vi "MWC.vi"() -> ()   [LabVIEW 2010]
doc: "This is the Target Temperature Monitoring module (TTM).\nIts job is to read all temperature measurement devices and report back the information."
panel:
  in  "Case Constant\n(See Context Help)":bool
  in  "Read HP":bool
  in  "Read FM":bool
  in  "Read Bellows":bool
  in  "Read EIP":bool=TRUE
  out "MWC Message Type":T1(ring)=enum."GenEvent="
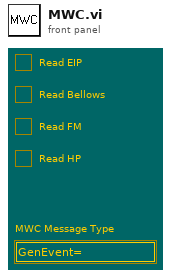
[diagram p1: front panel]
types:
  T1 = enum16{"Bad Message", "No Message", "FMAmplitude=", "FMOffset=", "Tune=", "Switch=", "GenEvent=", "Read", "Ping=", "Stop"}
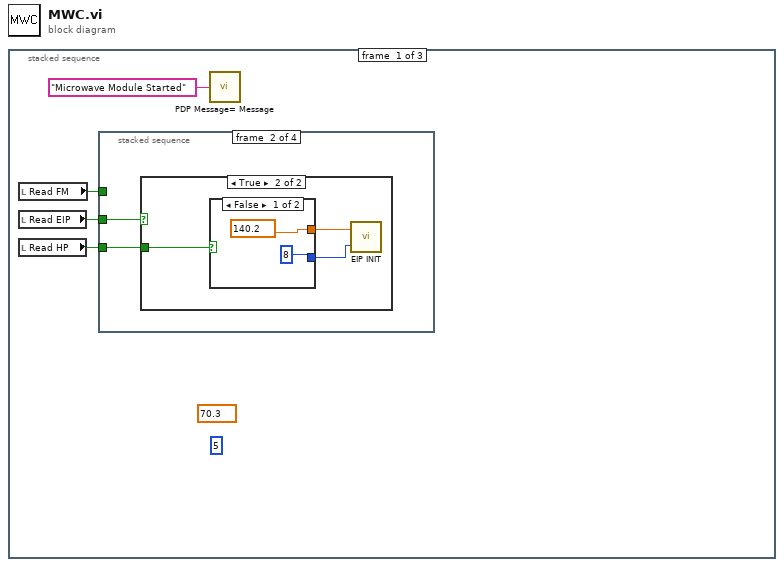
[diagram p0: block diagram]
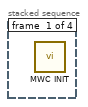
[diagram p2: hidden frame]
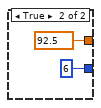
[diagram p4: hidden frame]
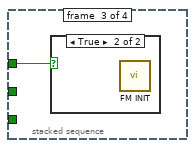
[diagram p5: hidden frame]
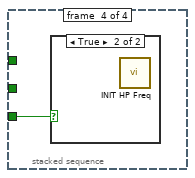
[diagram p7: hidden frame]
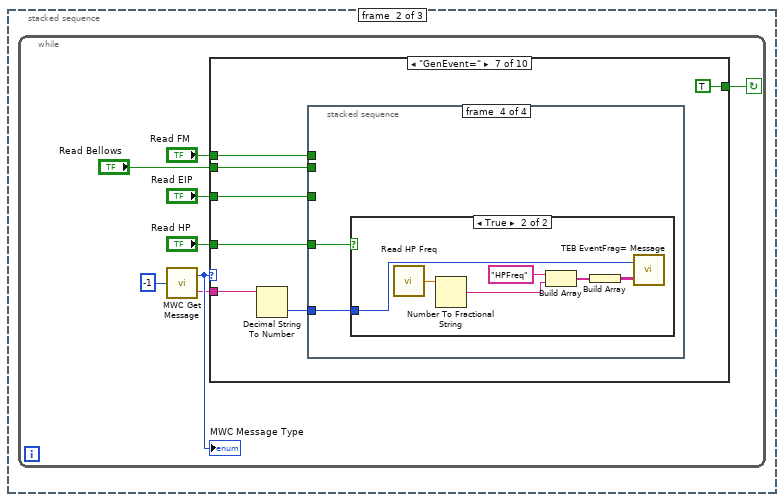
[diagram p9: hidden frame]
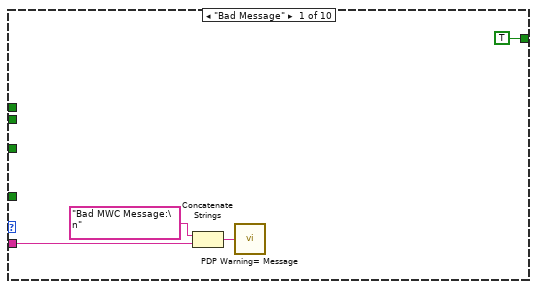
[diagram p10: hidden frame]
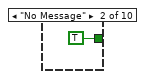
[diagram p11: hidden frame]
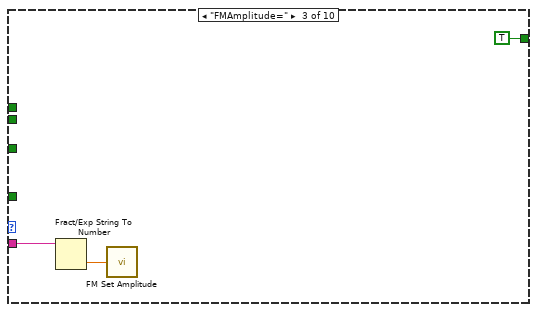
[diagram p12: hidden frame]
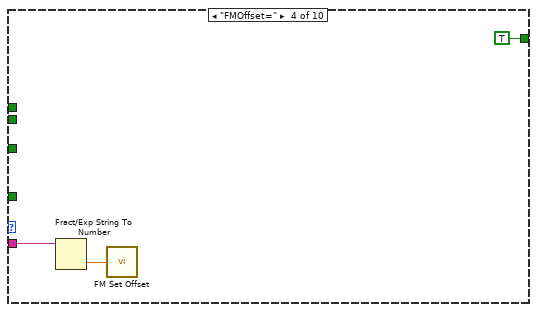
[diagram p13: hidden frame]
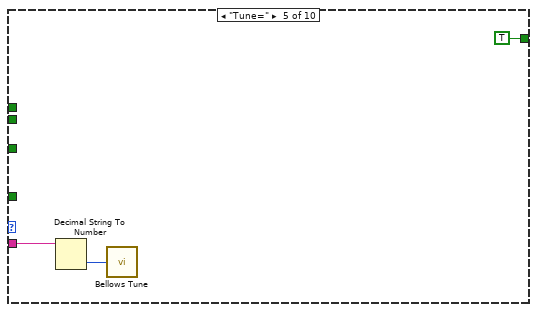
[diagram p14: hidden frame]
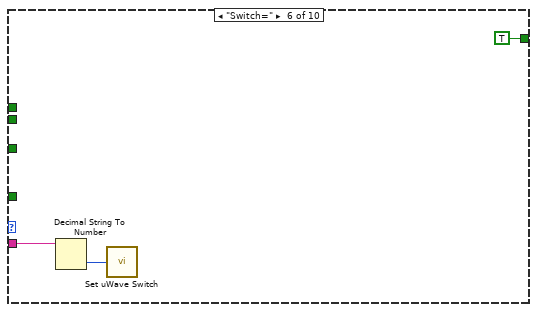
[diagram p15: hidden frame]
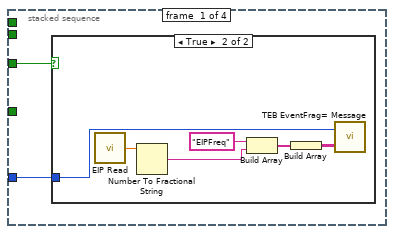
[diagram p16: hidden frame]
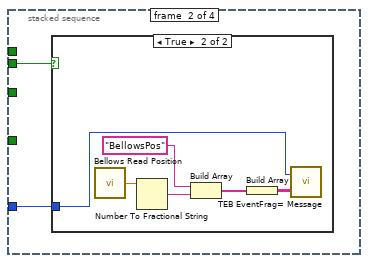
[diagram p18: hidden frame]
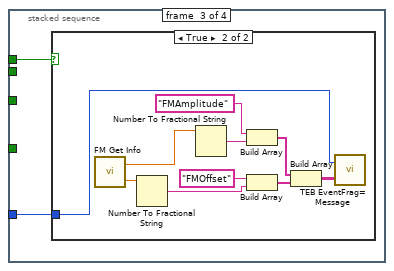
[diagram p20: hidden frame]
diagram:
  n1 = stacked-sequence {
    frame #0 {
      (unwired) 5 ("Subband")
      (unwired) 70.3 ("Center Freq (GHz)")
      n2 = local read "Read FM"() -> (w2:bool)
      n3 = local read "Read EIP"() -> (w1:bool)
      n4 = local read "Read HP"() -> (w3:bool)
      n5 = stacked-sequence {
        tunnel: w2 -> [_ _ w14 _]
        tunnel: w3 -> [_ w5 _ w15]
        tunnel: w1 -> [_ w6 _ _]
        frame #0 {
          n6 = call "MWC INIT.vi"() -> ()  [unwired: 1 in]
        }
        frame #1 {
          n7 = case shown="True" w6 {
            tunnel: w5 -> [_ w7]
            frame False {
            }
            frame True {
              n8 = case shown="False" w7 {
                tunnel: [140.2 ("Center Freq (GHz)") 92.5 ("Center Freq (GHz)")] -> w9
                tunnel: [8 ("Subband") 6 ("Subband")] -> w8
                frame False {
                }
                frame True {
                }
              }
              n9 = call "EIP INIT.vi"("Subband"=w8, "Center Freq (GHz)"=w9) -> ()
            }
          }
        }
        frame #2 {
          n10 = case shown="True" w14 {
            frame False {
            }
            frame True {
              n11 = call "FM INIT.vi"() -> ()  [unwired: 1 in]
            }
          }
        }
        frame #3 {
          n12 = case shown="True" w15 {
            frame False {
            }
            frame True {
              n13 = call "INIT HP Freq.vi"() -> ()  [unwired: 1 in]
            }
          }
        }
      }
      n14 = call "PDP Message= Message.vi"("Message"="Microwave Module Started") -> ()
    }
    frame #1 {
      n15 = while {
        stop <- w23 continue-if-true
        n16 = call "MWC Get Message.VI"("Timeout ms (-1)"=-1) -> ("MWC Message Type"=w22:T1, "Text"=w21:string)
        "MWC Message Type" <- w22
        n17 = case shown="\"GenEvent=\"" w22 {
          tunnel: w21 -> [w27 _ w30 w33 w36 w39 w47 _ w90 _]
          tunnel: [TRUE TRUE TRUE TRUE TRUE TRUE TRUE TRUE TRUE FALSE] -> w23
          tunnel: "Read EIP" -> [_ _ _ _ _ _ w44 _ _ _]
          tunnel: "Read Bellows" -> [_ _ _ _ _ _ w43 _ _ _]
          tunnel: "Read FM" -> [_ _ _ _ _ _ w42 _ _ _]
          tunnel: "Read HP" -> [_ _ _ _ _ _ w41 _ _ _]
          frame "Bad Message" {
            n18 = Concatenate Strings("Bad MWC Message:\n", w27) -> (w25:string)
            n19 = call "PDP Warning= Message.vi"("Message"=w25) -> ()
          }
          frame "No Message" {
          }
          frame "FMAmplitude=" {
            n20 = Fract/Exp String To Number(string=w30) -> (number=w29:dbl)  [unwired: 3 in, 1 out]
            n21 = call "FM Set Amplitude.vi"("Amplitude (V)"=w29) -> ()
          }
          frame "FMOffset=" {
            n22 = Fract/Exp String To Number(string=w33) -> (number=w32:dbl)  [unwired: 3 in, 1 out]
            n23 = call "FM Set Offset.vi"("Offset (V)"=w32) -> ()
          }
          frame "Tune=" {
            n24 = Decimal String To Number(string=w36) -> (number=w35:i32)  [unwired: 2 in, 1 out]
            n25 = call "Bellows Tune.vi"("Tune Amount"=w35) -> ()
          }
          frame "Switch=" {
            n26 = Decimal String To Number(string=w39) -> (number=w38:i32)  [unwired: 2 in, 1 out]
            n27 = call "Set uWave Switch.vi"("uWave Switch"=w38) -> ()
          }
          frame "GenEvent=" {
            n28 = Decimal String To Number(string=w47) -> (number=w45:i32)  [unwired: 2 in, 1 out]
            n29 = stacked-sequence {
              tunnel: w45 -> [w49 w57 w65 w77]
              tunnel: w44 -> [w48 _ _ _]
              tunnel: w43 -> [_ w56 _ _]
              tunnel: w42 -> [_ _ w64 _]
              tunnel: w41 -> [_ _ _ w76]
              frame #0 {
                n30 = case shown="True" w48 {
                  tunnel: w49 -> [_ w55]
                  frame False {
                  }
                  frame True {
                    n31 = call "EIP Read.vi"() -> ("Output"=w52:dbl)
                    n32 = Number To Fractional String(number=w52) -> (F-format string=w54:string)  [unwired: 3 in]
                    n33 = Build Array("EIPFreq", w54) -> (w51:string[])
                    n34 = Build Array(w51) -> (w50:string[][])
                    n35 = call "TEB EventFrag= Message.vi"("Event Fragment(s)"=w50, "Event Number"=w55) -> ()
                  }
                }
              }
              frame #1 {
                n36 = case shown="True" w56 {
                  tunnel: w57 -> [_ w63]
                  frame False {
                  }
                  frame True {
                    n37 = call "Bellows Read Position.vi"() -> ("Bellows Pos"=w61:dbl)
                    n38 = Number To Fractional String(number=w61) -> (F-format string=w60:string)  [unwired: 3 in]
                    n39 = Build Array("BellowsPos", w60) -> (w58:string[])
                    n40 = Build Array(w58) -> (w62:string[][])
                    n41 = call "TEB EventFrag= Message.vi"("Event Fragment(s)"=w62, "Event Number"=w63) -> ()
                  }
                }
              }
              frame #2 {
                n42 = case shown="True" w64 {
                  tunnel: w65 -> [_ w75]
                  frame False {
                  }
                  frame True {
                    n43 = call "FM Get Info.vi"() -> ("Offset (V)"=w68:dbl, "Amplitude (V)"=w71:dbl)
                    n44 = Number To Fractional String(number=w68) -> (F-format string=w70:string)  [unwired: 3 in]
                    n45 = Number To Fractional String(number=w71) -> (F-format string=w72:string)  [unwired: 3 in]
                    n46 = Build Array("FMAmplitude", w72) -> (w67:string[])
                    n47 = Build Array("FMOffset", w70) -> (w66:string[])
                    n48 = Build Array(w67, w66) -> (w74:string[][])
                    n49 = call "TEB EventFrag= Message.vi"("Event Fragment(s)"=w74, "Event Number"=w75) -> ()
                  }
                }
              }
              frame #3 {
                n50 = case shown="True" w76 {
                  tunnel: w77 -> [_ w83]
                  frame False {
                  }
                  frame True {
                    n51 = call "Read HP Freq.vi"() -> ("Frequency (GHz)"=w78:dbl)
                    n52 = Number To Fractional String(number=w78) -> (F-format string=w80:string)  [unwired: 3 in]
                    n53 = Build Array("HPFreq", w80) -> (w79:string[])
                    n54 = Build Array(w79) -> (w82:string[][])
                    n55 = call "TEB EventFrag= Message.vi"("Event Fragment(s)"=w82, "Event Number"=w83) -> ()
                  }
                }
              }
            }
          }
          frame "Read" {
            n56 = case shown="False" "Case Constant\n(See Context Help)" {
              frame False {
              }
              frame True {
                n57 = call "EIP Read.vi"() -> ("Output"=w86:dbl)
                n58 = call "PDP uWaveFreq= Message.vi"("uWave Freq"=w86) -> ()
              }
            }
          }
          frame "Ping=" {
            n59 = Get Date/Time In Seconds() -> (seconds since 1Jan1904=w87:timestamp)
            n60 = To Double Precision Float(number=w87) -> (double precision float=w91:dbl)
            n61 = Format Into String(format string="PingResponse=MWC,%.0f", w91) -> (resulting string=w89:string)  [unwired: 2 in, 1 out]
            n62 = call "Message Send.vi"("Message"=w89, "Destination"=w90) -> ()
          }
          frame "Stop" {
          }
        }
      }
    }
    frame #2 {
    }
  }
